vi "TCP.IP Client for Ripple Detection_requirements.vi"() -> ()   [LabVIEW 2021]
doc: "Demonstrates how to open a connection to an TCP server, read the data being sent, and display the data on a chart. This VI is designed to stop if the TCP connection is terminated."
uses:
  <vilib>/Analysis/3filter.llb/Filter Passband Type.ctl
  <vilib>/ptbypt/NI_PtbyPt.lvlib
  <vilib>/Analysis/NI_AALBase.lvlib
  <vilib>/Analysis/3filter.llb/Butterworth Filter (DBL).vi
panel:
  out "Array Size 2":u32
  out "error IO":errorcluster
  in  "File Name":path=path "F:/Career/Work/From Now/Book2.csv"
  out "Filtered":dbl[](graph)
  out "Array Size 3":u32
  out "Delayed RMS2>RMS1 for 3 data":dynamicdata(graph)
  out "RMS2>RMS1 for 3 data":dynamicdata(graph)
  out "Array Size":u32
  out "RMS2>RMS1":dynamicdata(graph)
  out "RMS1":dynamicdata(graph)
  out "RMS2":dynamicdata(graph)
  out "Raw Data Collected":dynamicdata(graph)
  in  "Boolean":bool
  in  "Server Closed":string="The server VI closed the connection."
  out "Raw Data":dbl[](graph)
  in  "Stop":bool
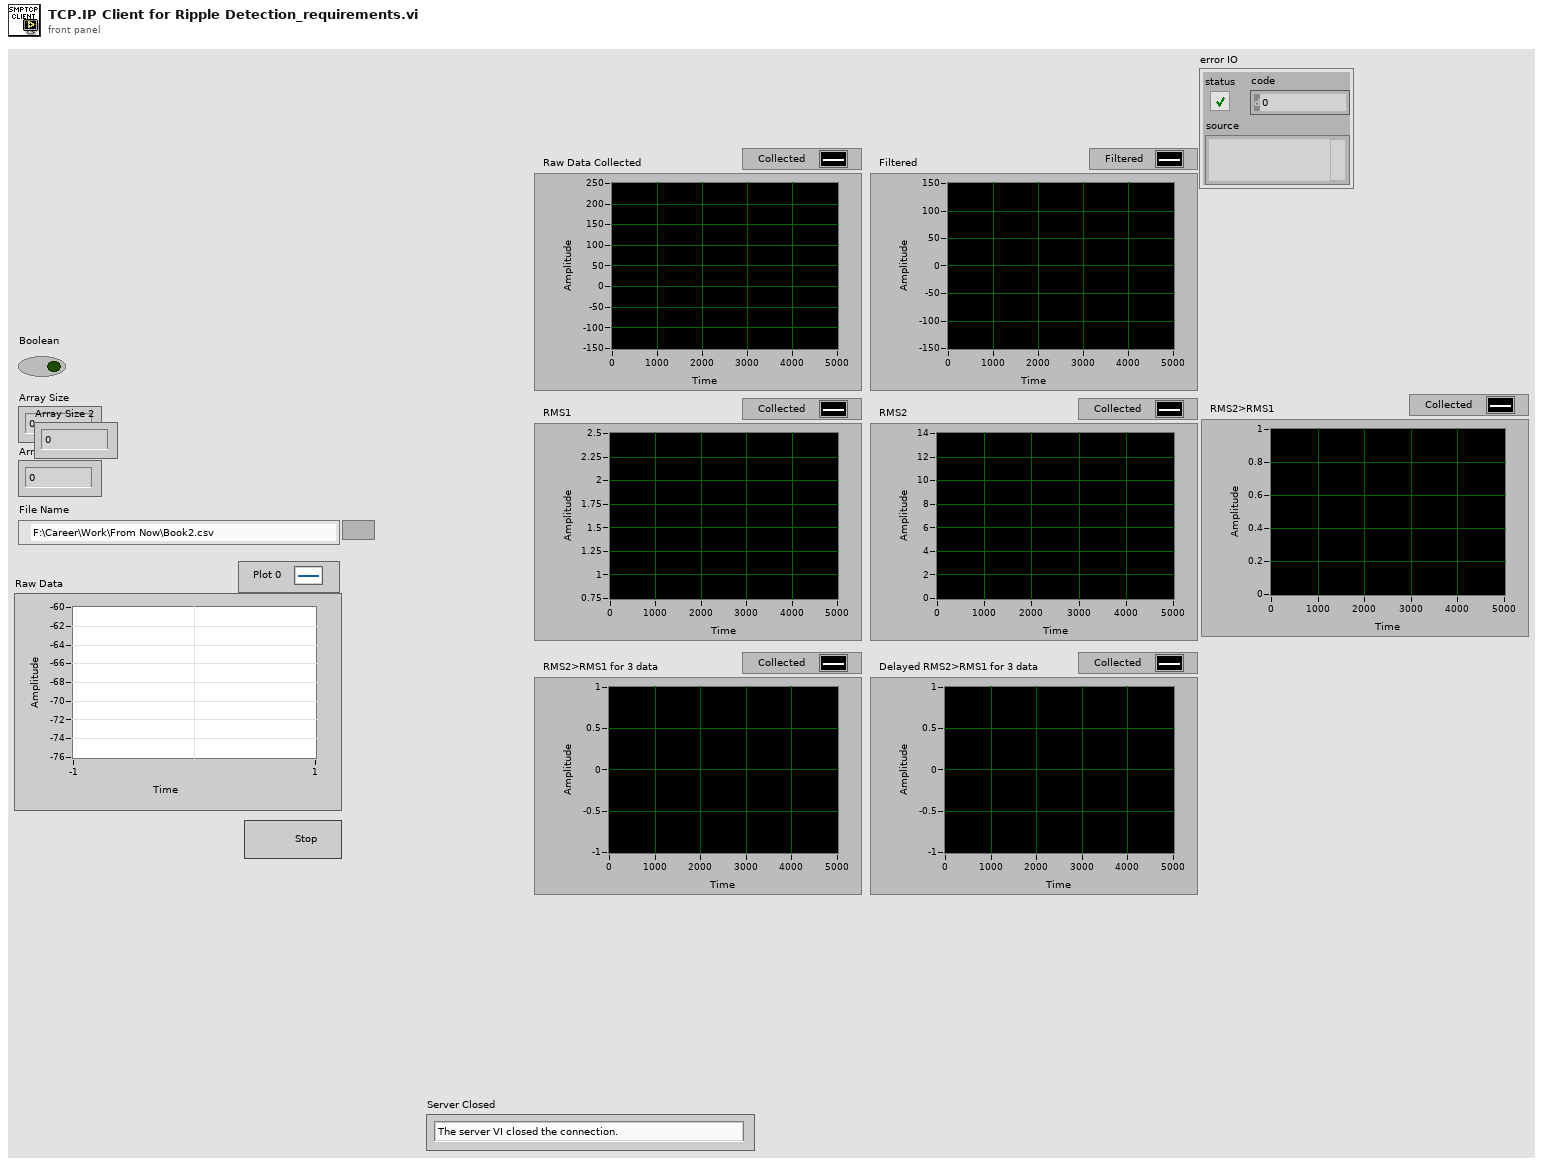
[diagram p1: front panel]
types:
  T1 = enum16{"open", "replace", "create", "open or create", "replace or create", "replace or create with confirmation"}
  T2 = typedef "NI_AALBase.lvlib/Filter Passband Type.ctl" = enum32{"Lowpass", "Highpass", "Bandpass", "Bandstop"}
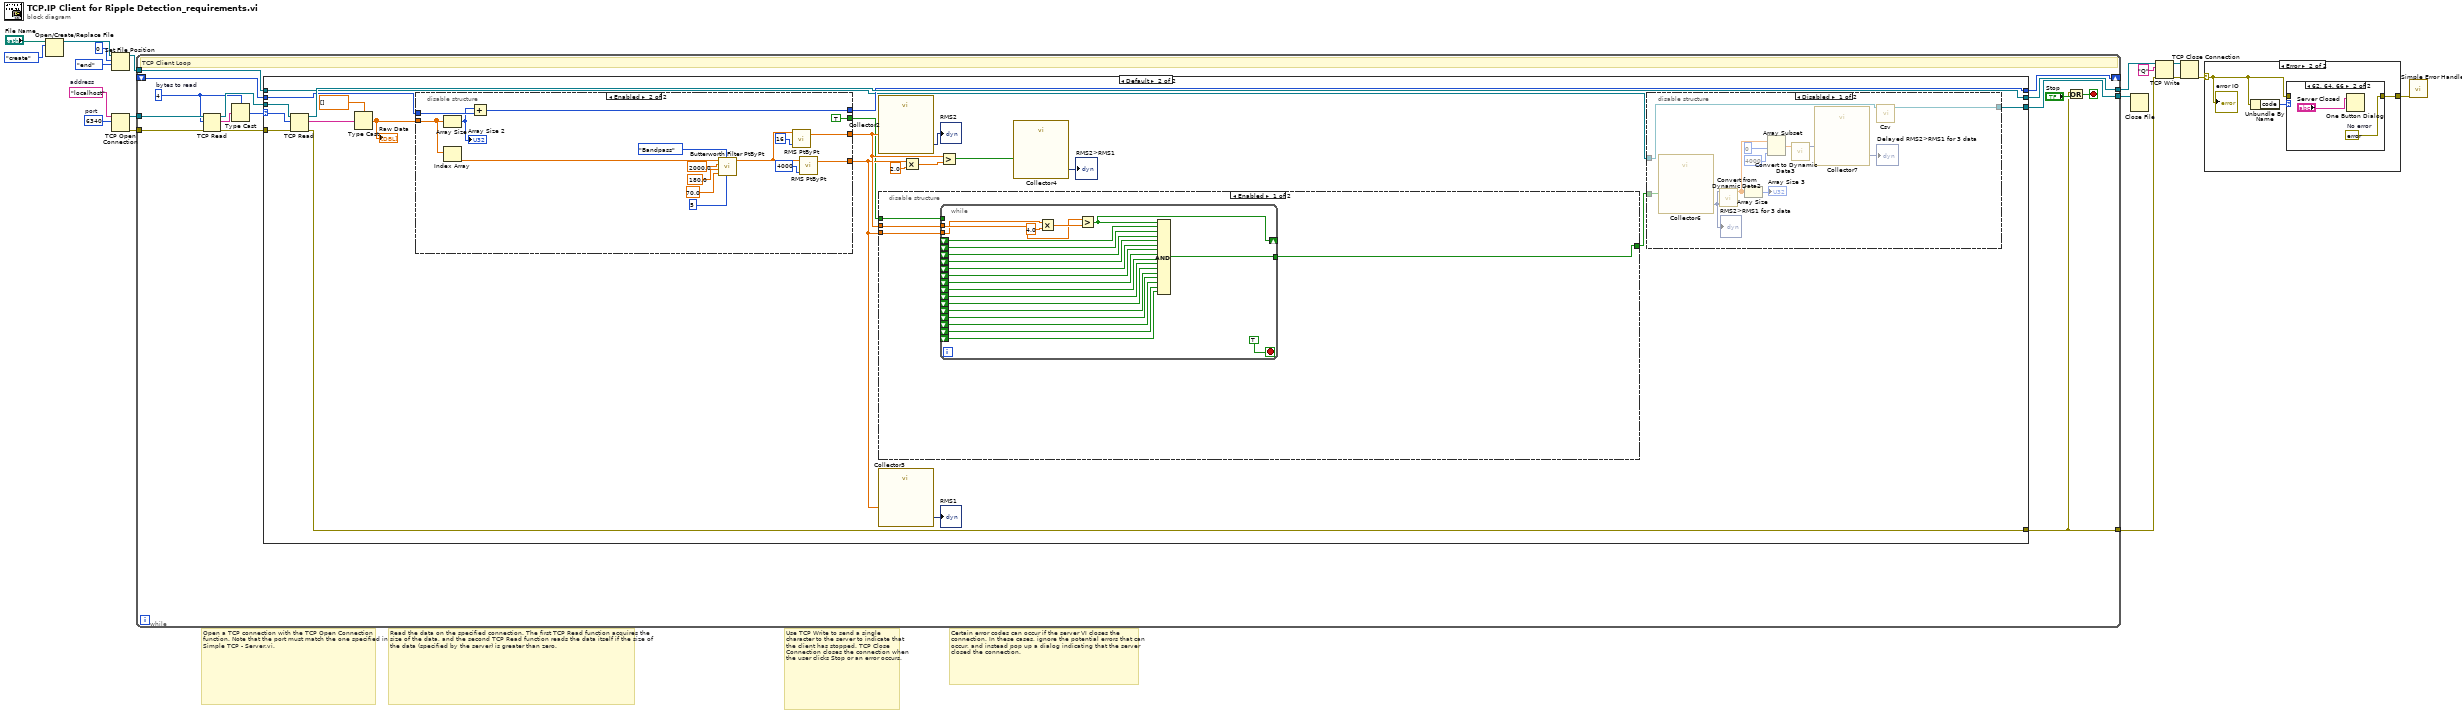
[diagram p0: block diagram]
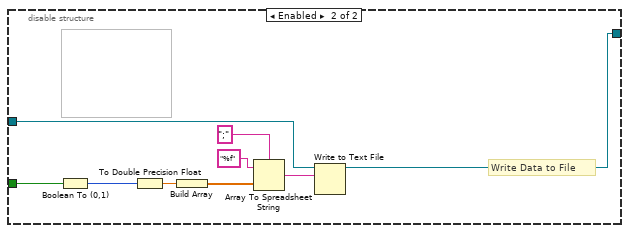
[diagram p5: hidden frame]
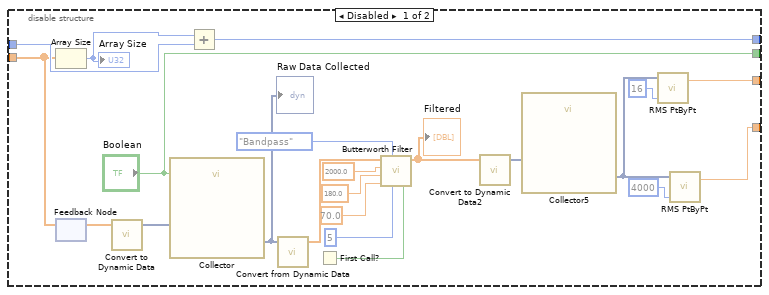
[diagram p6: hidden frame]
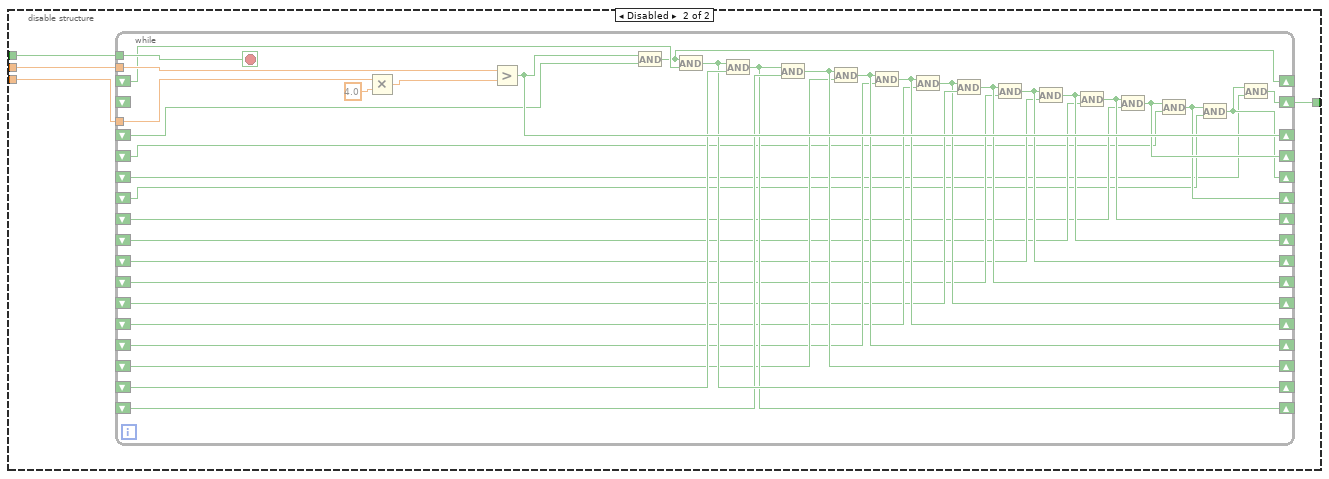
[diagram p7: hidden frame]
diagram:
  w1 = u16 6340  # port
  w9 = "localhost"  # address
  # "Certain error codes can occur if the server VI closes the connection. In these cases, ignore the potential errors that can occur, and instead pop up a dialog indicating that the server closed the connection."
  # "Use TCP Write to send a single character to the server to indicate that the client has stopped. TCP Close Connection closes the connection when the user clicks Stop or an error occurs."
  # "Read the data on the specified connection. The first TCP Read function acquires the size of the data, and the second TCP Read function reads the data itself if the size of the data (specified by the server) is greater than zero."
  # "Open a TCP connection with the TCP Open Connection function. Note that the port must match the one specified in Simple TCP - Server.vi."
  n1 = Open/Create/Replace File(file path (use dialog)="File Name", operation (0:open)=T1."create") -> (refnum out=w3:refnum<file>)  [unwired: 4 in, 2 out]
  n2 = Set File Position(offset (in bytes) (0)=i64 0, refnum=w3, from (0:start)=enum16{"start", "end", "current"}."end") -> (refnum out=w2:refnum<file>)  [unwired: 1 in, 1 out]
  n3 = TCP Open Connection(address=w9, remote port or service name=w1) -> (connection ID=w18:refnum<k5>, error out=w17:errorcluster)  [unwired: 3 in]
  n4 = while {
    tunnel: w17 -> [w29]
    tunnel: w18 -> [w30]
    tunnel: [w25] -> w15
    tunnel: [w24] -> w13
    shift-right: [w21] -> _
    shift-left: _ -> [w22]
    tunnel: [w20] -> w8
    tunnel: w2 -> [w19]
    stop <- w26 stop-if-true
    w28 = 4  # bytes to read
    # "TCP Client Loop"
    n5 = TCP Read(connection ID=w30, bytes to read=w28, error in (no error)=w29) -> (connection ID out=w32:refnum<k5>, data out=w33:string, error out=w31:errorcluster)  [unwired: 2 in]
    n6 = Type Cast(type=w28, x=w33) -> (*(type *) &x=w23:i32)
    n7 = case shown="Default" w23 {
      selector: w23 -> [_ w53]
      tunnel: w32 -> [w37 w59]
      tunnel: w31 -> [w36 w58]
      tunnel: [w37 w56] -> w25
      tunnel: [w36 w55] -> w24
      tunnel: w22 -> [w35 w49]
      tunnel: [w35 w48] -> w21
      tunnel: w19 -> [w34 w43]
      tunnel: [w34 w42] -> w20
      frame ..0 {
        # "The server has not written any data"
      }
      frame Default {
        n8 = TCP Read(connection ID=w59, bytes to read=w53, error in (no error)=w58) -> (connection ID out=w56:refnum<k5>, data out=w54:string, error out=w55:errorcluster)  [unwired: 2 in]
        n9 = Type Cast(type=dbl[] [] ("chart"), x=w54) -> (*(type *) &x=w47:dbl[])
        "Raw Data" <- w47
        n10 = disable-structure shown="Enabled" {
          disable-tunnel: [w100 w117] -> w52
          disable-tunnel: [w99 w116] -> w51
          disable-tunnel: ["Boolean" TRUE ("Enable")] -> w50
          disable-tunnel: w49 -> [w97 w115]
          disable-tunnel: [w96 w114] -> w48
          disable-tunnel: w47 -> [w95 w108]
          frame Disabled {
            n11 = Array Size(array=w95) -> (size(s)=w94:i32)
            "Array Size" <- w94
            n12 = feedback #1() -> (w87:dbl[])  [unwired: 1 in]
            n13 = feedback-in #1(w95) -> ()
            n14 = call "Convert to Dynamic Data"("Array"=w87) -> ("Dynamic Data Type"=w88:dynamicdata)  [unwired: 3 in]
            n15 = call "Collector"("Enable"="Boolean", "Signals"=w88) -> ("Collected Signals"=w101:dynamicdata)  [unwired: 8 in, 1 out]
            "Raw Data Collected" <- w101
            n16 = Add(x=w94, y=w97) -> (x+y=w96:i32)
            n17 = call "Convert from Dynamic Data"("Dynamic Data Type"=w101) -> ("Array"=w89:dbl[])  [unwired: 3 in]
            n18 = First Call?() -> (First Call?: T/F=w80:bool)
            n19 = call-poly <vilib>:"Butterworth Filter.vi"("init/cont (init:F)"=w80, "order"=5, "filter type"=Filter_Passband_Type."Bandpass", "low cutoff freq: fl"=70.0, "high cutoff freq: fh"=180.0, "sampling freq: fs"=2000.0, "X"=w89) -> ("Filtered X"=w93:dbl[])  [unwired: 1 in, 1 out]
            "Filtered" <- w93
            n20 = call "Convert to Dynamic Data2"("Array"=w93) -> ("Dynamic Data Type"=w84:dynamicdata)  [unwired: 3 in]
            n21 = call "Collector5"("Signals"=w84) -> ("Collected Signals"=w83:dynamicdata)  [unwired: 9 in, 1 out]
            n22 = call <vilib>:"RMS PtByPt.vi"("sample length"=16, "x"=w83) -> ("rms value"=w100:dbl)  [unwired: 2 in, 1 out]
            n23 = call <vilib>:"RMS PtByPt.vi"("sample length"=4000, "x"=w83) -> ("rms value"=w99:dbl)  [unwired: 2 in, 1 out]
          }
          frame Enabled {
            n24 = Array Size(array=w108) -> (size(s)=w113:i32)
            "Array Size 2" <- w113
            n25 = Index Array(array=w108) -> (element=w107:dbl)  [unwired: 1 in]
            n26 = Add(x=w113, y=w115) -> (x+y=w114:i32)
            n27 = call <vilib>:"Butterworth Filter PtByPt.vi"("order"=5, "filter type"=Filter_Passband_Type."Bandpass", "low cutoff freq: fl"=70.0, "high cutoff freq: fh"=180.0, "sampling freq: fs"=2000.0, "x"=w107) -> ("Filtered x"=w102:dbl)  [unwired: 3 in, 1 out]
            n28 = call <vilib>:"RMS PtByPt.vi"("sample length"=16, "x"=w102) -> ("rms value"=w117:dbl)  [unwired: 2 in, 1 out]
            n29 = call <vilib>:"RMS PtByPt.vi"("sample length"=4000, "x"=w102) -> ("rms value"=w116:dbl)  [unwired: 2 in, 1 out]
          }
        }
        n30 = call "Collector2"("Signals"=w52) -> ("Collected Signals"=→"RMS2":dynamicdata)  [unwired: 9 in, 1 out]
        n31 = disable-structure shown="Enabled" {
          disable-tunnel: w52 -> [w121 w147]
          disable-tunnel: w51 -> [w120 w146]
          disable-tunnel: w50 -> [w119 w145]
          disable-tunnel: [w118 w144] -> w38
          frame Enabled {
            n32 = while {
              tunnel: w121 -> [w141]
              tunnel: w120 -> [w140]
              shift-right: [w123] -> _
              shift-left: _ -> [w124]
              tunnel: w119 -> [_]
              shift-left: _ -> [w125]
              shift-left: _ -> [w126]
              shift-left: _ -> [w127]
              shift-left: _ -> [w128]
              shift-left: _ -> [w129]
              shift-left: _ -> [w130]
              shift-left: _ -> [w131]
              shift-left: _ -> [w132]
              shift-left: _ -> [w133]
              shift-left: _ -> [w134]
              shift-left: _ -> [w135]
              tunnel: [w139] -> w118
              shift-left: _ -> [w136]
              shift-left: _ -> [w137]
              shift-left: _ -> [w138]
              stop <- TRUE stop-if-true
              n33 = Multiply(x=w140, y=4.0) -> (x*y=w142:dbl)
              n34 = Greater?(x=w141, y=w142) -> (0:w123:bool)
              n35 = Compound Arithmetic op=AND(w123, w124, w125, w126, w127, w128, w129, w130, w131, w132, w133, w134, w135, w136, w137, w138) -> (w139:bool)
            }
          }
          frame Disabled {
            n36 = while {
              tunnel: w147 -> [w181]
              tunnel: w146 -> [w180]
              shift-right: [w175] -> _
              shift-left: _ -> [w176]
              shift-right: [w178] -> _
              shift-left: _ -> [w177]
              tunnel: w145 -> [w179]
              shift-right: [w173] -> _
              shift-left: _ -> [w174]
              shift-right: [w171] -> _
              shift-left: _ -> [w172]
              shift-right: [w170] -> _
              shift-left: _ -> [w169]
              shift-right: [w161] -> _
              shift-left: _ -> [w154]
              shift-right: [w166] -> _
              shift-left: _ -> [w165]
              shift-right: [w168] -> _
              shift-left: _ -> [w167]
              shift-right: [w163] -> _
              shift-left: _ -> [w164]
              shift-right: [w162] -> _
              shift-left: _ -> [w155]
              shift-right: [w160] -> _
              shift-left: _ -> [w153]
              shift-right: [w159] -> _
              shift-left: _ -> [w152]
              shift-right: [w158] -> _
              shift-left: _ -> [w151]
              shift-right: [w157] -> _
              shift-left: _ -> [w150]
              shift-right: [w156] -> _
              shift-left: _ -> [w149]
              shift-right: [w148] -> w144
              shift-left: _ -> [_]
              stop <- w179 stop-if-true
              n37 = Multiply(x=w180, y=4.0) -> (x*y=w182:dbl)
              n38 = Greater?(x=w181, y=w182) -> (0:w178:bool)
              n39 = And(x=w178, y=w177) -> (x .and. y?=w175:bool)
              n40 = And(x=w175, y=w176) -> (x .and. y?=w173:bool)
              n41 = And(x=w173, y=w174) -> (x .and. y?=w171:bool)
              n42 = And(x=w171, y=w172) -> (x .and. y?=w170:bool)
              n43 = And(x=w170, y=w169) -> (x .and. y?=w168:bool)
              n44 = And(x=w168, y=w167) -> (x .and. y?=w166:bool)
              n45 = And(x=w166, y=w165) -> (x .and. y?=w163:bool)
              n46 = And(x=w163, y=w164) -> (x .and. y?=w162:bool)
              n47 = And(x=w162, y=w155) -> (x .and. y?=w161:bool)
              n48 = And(x=w161, y=w154) -> (x .and. y?=w160:bool)
              n49 = And(x=w160, y=w153) -> (x .and. y?=w159:bool)
              n50 = And(x=w159, y=w152) -> (x .and. y?=w158:bool)
              n51 = And(x=w158, y=w151) -> (x .and. y?=w157:bool)
              n52 = And(x=w157, y=w150) -> (x .and. y?=w156:bool)
              n53 = And(x=w156, y=w149) -> (x .and. y?=w148:bool)
            }
          }
        }
        n54 = call "Collector3"("Signals"=w51) -> ("Collected Signals"=→"RMS1":dynamicdata)  [unwired: 9 in, 1 out]
        n55 = Multiply(x=w51, y=2.0) -> (x*y=w40:dbl)
        n56 = Greater?(x=w52, y=w40) -> (0:w39:bool)
        n57 = call "Collector4"("Signals"=w39) -> ("Collected Signals"=→"RMS2>RMS1":dynamicdata)  [unwired: 9 in, 1 out]
        n58 = disable-structure shown="Disabled" {
          disable-tunnel: w43 -> [w67 w76]
          disable-tunnel: [w66 w75] -> w42
          disable-tunnel: w38 -> [w60 w74]
          frame Disabled {
            n59 = call "Collector6"("Signals"=w60) -> ("Collected Signals"=w70:dynamicdata)  [unwired: 9 in, 1 out]
            "RMS2>RMS1 for 3 data" <- w70
            n60 = call "Convert from Dynamic Data2"("Dynamic Data Type"=w70) -> ("Array"=w62:dbl[])  [unwired: 3 in]
            n61 = Array Size(array=w62) -> (size(s)=→"Array Size 3":i32)
            n62 = Array Subset(array=w62, index=0, length=4000 ("index")) -> (w61:dbl[])
            n63 = call "Convert to Dynamic Data3"("Array"=w61) -> ("Dynamic Data Type"=w65:dynamicdata)  [unwired: 3 in]
            n64 = call "Collector7"("Signals"=w65) -> ("Collected Signals"=→"Delayed RMS2>RMS1 for 3 data":dynamicdata)  [unwired: 9 in, 1 out]
            n65 = call "Csv.vi"("Byte Stream File in"=w67) -> ("Byte Stream File out"=w66:refnum<file>)  [unwired: 10 in]
          }
          frame Enabled {
            # "Write Data to File"
            n66 = Boolean To (0,1)(Boolean=w74) -> (0, 1=w73:i16)
            n67 = To Double Precision Float(number=w73) -> (double precision float=w72:dbl)
            n68 = Build Array(w72) -> (w71:dbl[])
            n69 = Array To Spreadsheet String(delimiter (Tab)=";" ("delimiter (\\t)"), array=w71, 3:"%f" ("format string")) -> (spreadsheet string=w77:string)
            n70 = Write to Text File(file (use dialog)=w76, text=w77) -> (refnum out=w75:refnum<file>)  [unwired: 2 in, 2 out]
          }
        }
      }
    }
    n71 = Or(x=w24, y="Stop") -> (x .or. y?=w26:bool)
  }
  n72 = Close File(refnum=w8) -> ()  [unwired: 1 in, 2 out]
  n73 = TCP Write(connection ID=w15, data in="Q", error in (no error)=w13) -> (connection ID out=w16:refnum<k5>, error out=w14:errorcluster)  [unwired: 2 out]
  n74 = TCP Close Connection(connection ID=w16, error in (no error)=w14) -> (error out=w11:errorcluster)  [unwired: 1 in, 1 out]
  n75 = case shown="Error" w11 {
    selector: w11 -> [w184 w185]
    tunnel: [w184 w186] -> w10
    frame No Error {
    }
    frame Error {
      n76 = Unbundle By Name(w185) -> ("code"=w187:i32)
      n77 = case shown="62, 64, 66" w187 {
        tunnel: w185 -> [w188 _]
        tunnel: [w188 w190] -> w186
        frame Default {
        }
        frame 62, 64, 66 {
          w190 = errorcluster {"status"=FALSE, "code"=0, "source"=""}  # No error
          n78 = One Button Dialog(message="Server Closed") -> ()  [unwired: 1 in, 1 out]
        }
      }
      "error IO" <- w185
    }
  }
  n79 = call <vilib>:"Simple Error Handler.vi"("error in (no error)"=w10) -> ()  [unwired: 4 in, 5 out]
